vi "Get IC Array Size.vi"(8 "error in (no error)":errorcluster, 11 "PDE_Wave_1D in":refnum<class "NI_PDE_Wave_1D.lvclass">) -> (0 "error out":errorcluster, 2 "# of IC":i32, 3 "PDE_Wave_1D out":refnum<class "NI_PDE_Wave_1D.lvclass">)   [LabVIEW 2017, in "NI_PDE.lvlib" / "NI_PDE_Wave_1D.lvclass"]
uses:
  <vilib>/gmath/pde.llb/PDEClass/PDE_Wave_1D/NI_PDE_Wave_1D.lvclass
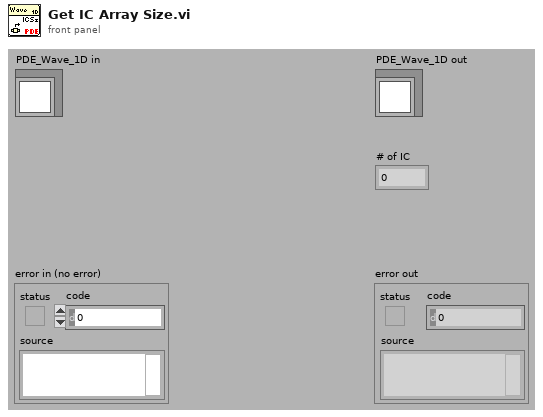
[diagram p1: front panel]
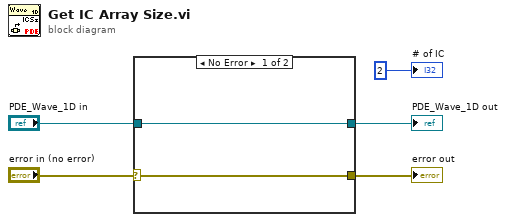
[diagram p0: block diagram]
diagram:
  n1 = case shown="No Error" "error in (no error)" {
    selector: "error in (no error)" -> [w6 w9]
    tunnel: "PDE_Wave_1D in" -> [w7 w8]
    tunnel: [w7 w8] -> w4
    tunnel: [w6 w9] -> w3
    frame No Error {
    }
    frame Error {
    }
  }
  "PDE_Wave_1D out" <- w4
  "error out" <- w3
  "# of IC" <- 2 ("# of IC")
